vi "LC-MISDK_SimpleInjector.ActivationException.vi"() -> ()   [LabVIEW 2015]
uses:
  C:/Program Files (x86)/National Instruments/LabVIEW 2015/LC-MISDK.dll
  Program Files (x86)/National Instruments/LabVIEW 2015/LC-MISDK.dll
panel:
  out "X":dbl
  out "Y":dbl
  out "Z":dbl
  out "Lv":dbl
  out "Dw":dbl
  out "Pe":dbl
  out "Lv":dbl
  out "Tcp":dbl
  out "Duv":dbl
  out "ReadLatestData Error":dbl format="%#_6f"
  out "Lv":dbl
  out "ud":dbl
  out "vd":dbl
  in  "Get Measurement Data":T1(radio)=enum."Lvxy"
  in  "Measurement":bool
  out "y":dbl
  out "x":dbl
  out "Lv":dbl
  out "Connect error Code":dbl
  in  "EXIT":bool
  in  "Connect":bool
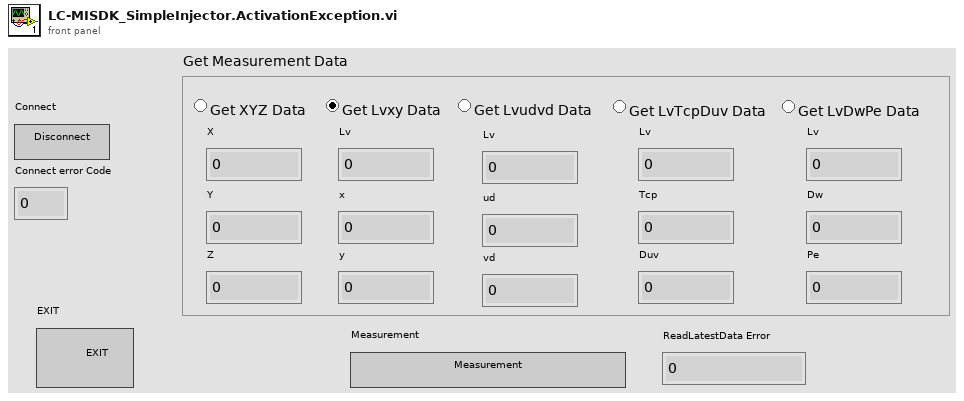
[diagram p1: front panel]
types:
  T1 = enum32{"XYZ", "Lvxy", "Lvudvd", "LvTcpDuv", "LvDwPe"}
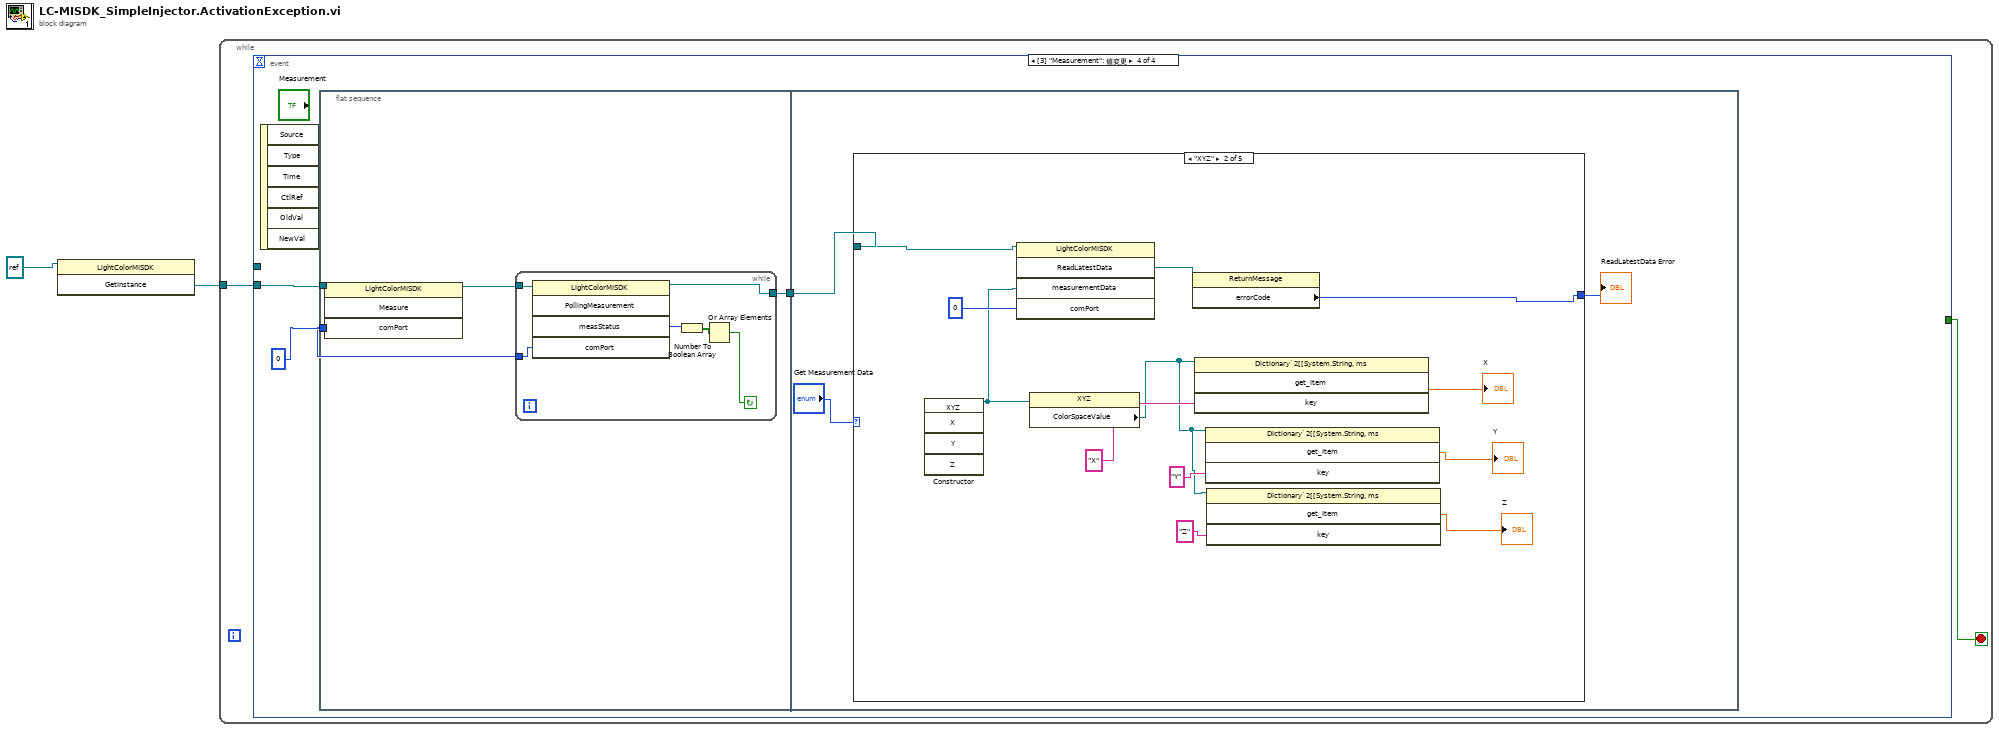
[diagram p0: block diagram]
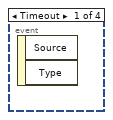
[diagram p2: hidden frame]
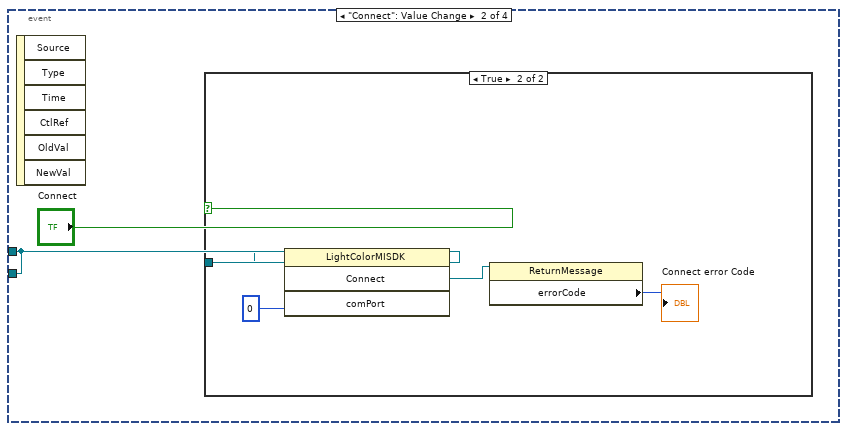
[diagram p3: hidden frame]
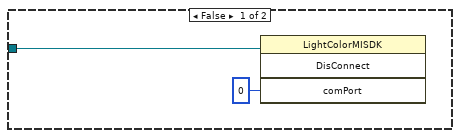
[diagram p4: hidden frame]
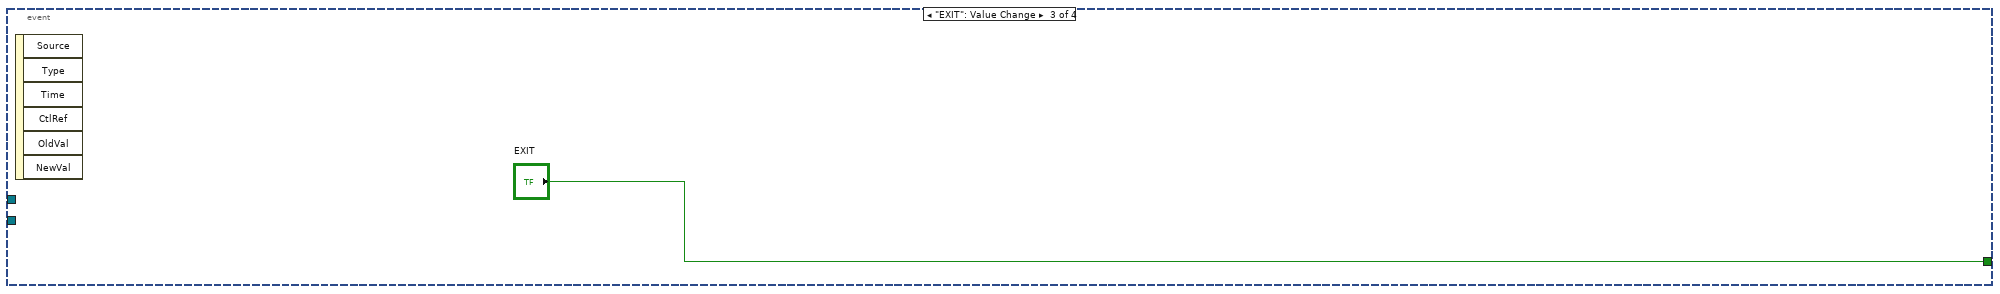
[diagram p5: hidden frame]
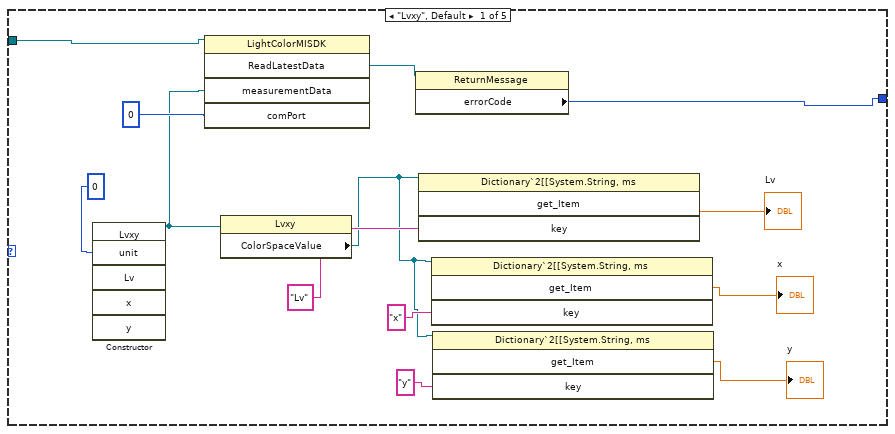
[diagram p6: hidden frame]
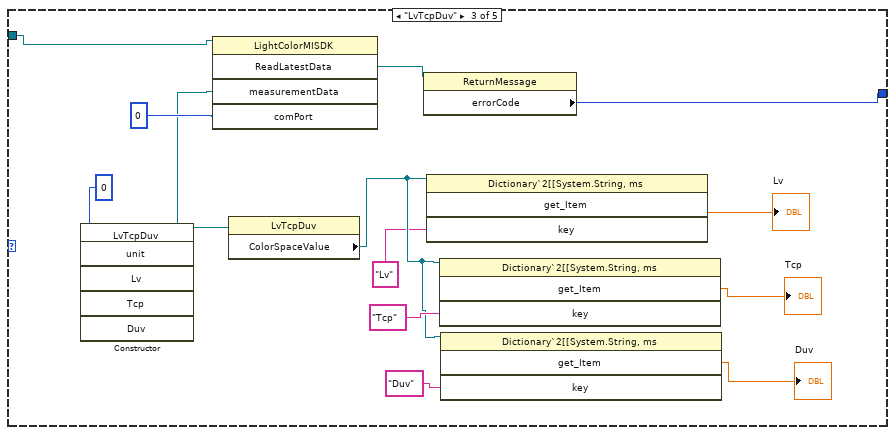
[diagram p7: hidden frame]
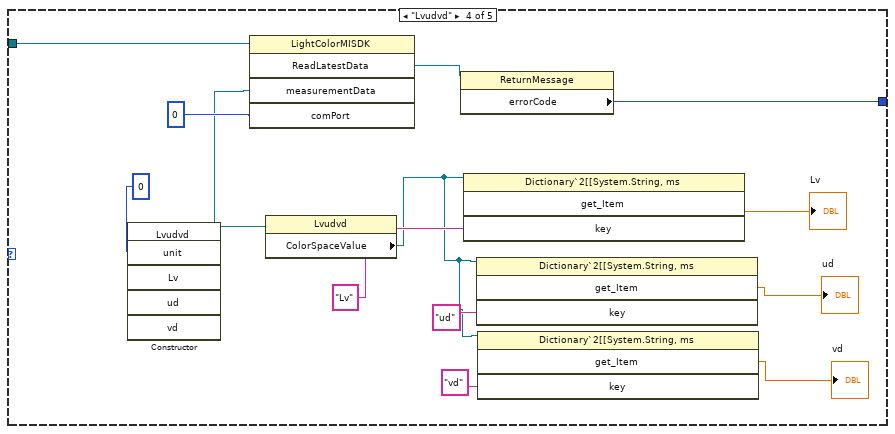
[diagram p8: hidden frame]
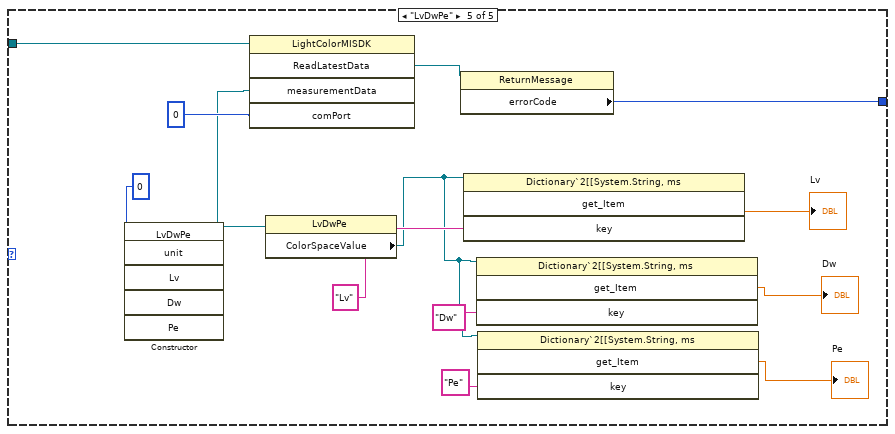
[diagram p9: hidden frame]
diagram:
  n1 = invoke on="インボークノード" class="LightColorMISDK" method="GetInstance"(reference=refnum<k24> refnum ("リファレンス出力")) -> ("GetInstance"=w1:refnum<k24>)  [unwired: 2 in, 2 out]
  n2 = while {
    tunnel: w1 -> [w4]
    stop <- w3 stop-if-true
    n3 = event shown="[3] \"Measurement\": 値変更" {
      selector: _ -> [_ _ _ _]
      dyn-events: _ -> [_ _ _ _]
      timeout: _ -> [_ _ _ _]
      tunnel: [_ w5 _ _] -> _
      tunnel: [_ _ "EXIT" _] -> w3
      tunnel: w4 -> [_ w5 _ w16]
      event Timeout {
        n4 = event-data() -> ()  [unwired: 1 in, 2 out]
      }
      event "Connect": Value Change {
        n5 = event-data() -> ()  [unwired: 1 in, 6 out]
        n6 = case shown="TRUE" "Connect" {
          tunnel: w5 -> [w7 w12]
          frame False {
            n7 = invoke on="インボークノード" class="LightColorMISDK" method="DisConnect"(reference=w7, "comPort"=0) -> ()  [unwired: 2 in, 4 out]
          }
          frame True {
            n8 = invoke on="インボークノード" class="LightColorMISDK" method="Connect"(reference=w12, "comPort"=0) -> ("Connect"=w9:refnum<k24>)  [unwired: 2 in, 3 out]
            n9 = property on="プロパティノード" class="ReturnMessage"(reference=w9) -> ("errorCode"=→"Connect error Code":i32)  [unwired: 1 in, 2 out]
          }
        }
      }
      event "EXIT": Value Change {
        n10 = event-data() -> ()  [unwired: 1 in, 6 out]
      }
      event "Measurement": Value Change {
        n11 = event-data() -> ()  [unwired: 1 in, 6 out]
        n12 = flat-sequence {
          tunnel: w16 -> [w19]
          tunnel: 0 -> [w17]
          tunnel: [w20] -> w14
          tunnel: w14 -> [w28]
          frame #0 {
            n13 = invoke on="インボークノード" class="LightColorMISDK" method="Measure"(reference=w19, "comPort"=w17) -> (reference out=w18:refnum<k24>)  [unwired: 2 in, 3 out]
            n14 = while {
              tunnel: [w25] -> w20
              tunnel: w18 -> [w24]
              tunnel: w17 -> [w23]
              stop <- w21 continue-if-true
              n15 = invoke on="インボークノード" class="LightColorMISDK" method="PollingMeasurement"(reference=w24, "comPort"=w23) -> (reference out=w25:refnum<k24>, "measStatus"=w26:i32)  [unwired: 3 in, 3 out]
              n16 = Number To Boolean Array(number=w26) -> (Boolean array=w22:bool[])
              n17 = Or Array Elements(Boolean array=w22) -> (logical OR=w21:bool)
            }
          }
          frame #1 {
            n18 = case shown="\"XYZ\"" "Get Measurement Data" {
              tunnel: w28 -> [w42 w54 w67 w80 w93]
              tunnel: [w30 w43 w55 w68 w81] -> w27
              frame "Lvxy", Default {
                n19 = constructor class="Lvxy"("unit"=0) -> (reference out=w39:refnum<k24>)  [unwired: 6 in, 6 out]
                n20 = invoke on="インボークノード" class="LightColorMISDK" method="ReadLatestData"(reference=w42, "measurementData"=w39, "comPort"=0) -> ("ReadLatestData"=w40:refnum<k24>)  [unwired: 2 in, 4 out]
                n21 = property class="Lvxy"(reference=w39) -> ("ColorSpaceValue"=w34:refnum<k24>)  [unwired: 1 in, 2 out]
                n22 = property on="プロパティノード" class="ReturnMessage"(reference=w40) -> ("errorCode"=w30:i32)  [unwired: 1 in, 2 out]
                n23 = invoke class="Dictionary`2[[System.String, ms" method="get_Item"(reference=w34, "key"="Lv") -> ("get_Item"=→"Lv":dbl)  [unwired: 2 in, 3 out]
                n24 = invoke class="Dictionary`2[[System.String, ms" method="get_Item"(reference=w34, "key"="x") -> ("get_Item"=→"x":dbl)  [unwired: 2 in, 3 out]
                n25 = invoke class="Dictionary`2[[System.String, ms" method="get_Item"(reference=w34, "key"="y") -> ("get_Item"=→"y":dbl)  [unwired: 2 in, 3 out]
              }
              frame "XYZ" {
                n26 = constructor class="XYZ"() -> (reference out=w51:refnum<k24>)  [unwired: 6 in, 5 out]
                n27 = invoke on="インボークノード" class="LightColorMISDK" method="ReadLatestData"(reference=w54, "measurementData"=w51, "comPort"=0) -> ("ReadLatestData"=w52:refnum<k24>)  [unwired: 2 in, 4 out]
                n28 = property class="XYZ"(reference=w51) -> ("ColorSpaceValue"=w46:refnum<k24>)  [unwired: 1 in, 2 out]
                n29 = property on="プロパティノード" class="ReturnMessage"(reference=w52) -> ("errorCode"=w43:i32)  [unwired: 1 in, 2 out]
                n30 = invoke class="Dictionary`2[[System.String, ms" method="get_Item"(reference=w46, "key"="X") -> ("get_Item"=→"X":dbl)  [unwired: 2 in, 3 out]
                n31 = invoke class="Dictionary`2[[System.String, ms" method="get_Item"(reference=w46, "key"="Y") -> ("get_Item"=→"Y":dbl)  [unwired: 2 in, 3 out]
                n32 = invoke class="Dictionary`2[[System.String, ms" method="get_Item"(reference=w46, "key"="Z") -> ("get_Item"=→"Z":dbl)  [unwired: 2 in, 3 out]
              }
              frame "LvTcpDuv" {
                n33 = constructor class="LvTcpDuv"("unit"=0) -> (reference out=w64:refnum<k24>)  [unwired: 6 in, 6 out]
                n34 = invoke on="インボークノード" class="LightColorMISDK" method="ReadLatestData"(reference=w67, "measurementData"=w64, "comPort"=0) -> ("ReadLatestData"=w65:refnum<k24>)  [unwired: 2 in, 4 out]
                n35 = property class="LvTcpDuv"(reference=w64) -> ("ColorSpaceValue"=w60:refnum<k24>)  [unwired: 1 in, 2 out]
                n36 = property on="プロパティノード" class="ReturnMessage"(reference=w65) -> ("errorCode"=w55:i32)  [unwired: 1 in, 2 out]
                n37 = invoke class="Dictionary`2[[System.String, ms" method="get_Item"(reference=w60, "key"="Lv") -> ("get_Item"=→"Lv":dbl)  [unwired: 2 in, 3 out]
                n38 = invoke class="Dictionary`2[[System.String, ms" method="get_Item"(reference=w60, "key"="Tcp") -> ("get_Item"=→"Tcp":dbl)  [unwired: 2 in, 3 out]
                n39 = invoke class="Dictionary`2[[System.String, ms" method="get_Item"(reference=w60, "key"="Duv") -> ("get_Item"=→"Duv":dbl)  [unwired: 2 in, 3 out]
              }
              frame "Lvudvd" {
                n40 = constructor class="Lvudvd"("unit"=0) -> (reference out=w77:refnum<k24>)  [unwired: 6 in, 6 out]
                n41 = invoke on="インボークノード" class="LightColorMISDK" method="ReadLatestData"(reference=w80, "measurementData"=w77, "comPort"=0) -> ("ReadLatestData"=w78:refnum<k24>)  [unwired: 2 in, 4 out]
                n42 = property class="Lvudvd"(reference=w77) -> ("ColorSpaceValue"=w72:refnum<k24>)  [unwired: 1 in, 2 out]
                n43 = property on="プロパティノード" class="ReturnMessage"(reference=w78) -> ("errorCode"=w68:i32)  [unwired: 1 in, 2 out]
                n44 = invoke class="Dictionary`2[[System.String, ms" method="get_Item"(reference=w72, "key"="Lv") -> ("get_Item"=→"Lv":dbl)  [unwired: 2 in, 3 out]
                n45 = invoke class="Dictionary`2[[System.String, ms" method="get_Item"(reference=w72, "key"="ud") -> ("get_Item"=→"ud":dbl)  [unwired: 2 in, 3 out]
                n46 = invoke class="Dictionary`2[[System.String, ms" method="get_Item"(reference=w72, "key"="vd") -> ("get_Item"=→"vd":dbl)  [unwired: 2 in, 3 out]
              }
              frame "LvDwPe" {
                n47 = constructor class="LvDwPe"("unit"=0) -> (reference out=w90:refnum<k24>)  [unwired: 6 in, 6 out]
                n48 = invoke on="インボークノード" class="LightColorMISDK" method="ReadLatestData"(reference=w93, "measurementData"=w90, "comPort"=0) -> ("ReadLatestData"=w91:refnum<k24>)  [unwired: 2 in, 4 out]
                n49 = property class="LvDwPe"(reference=w90) -> ("ColorSpaceValue"=w85:refnum<k24>)  [unwired: 1 in, 2 out]
                n50 = property on="プロパティノード" class="ReturnMessage"(reference=w91) -> ("errorCode"=w81:i32)  [unwired: 1 in, 2 out]
                n51 = invoke class="Dictionary`2[[System.String, ms" method="get_Item"(reference=w85, "key"="Lv") -> ("get_Item"=→"Lv":dbl)  [unwired: 2 in, 3 out]
                n52 = invoke class="Dictionary`2[[System.String, ms" method="get_Item"(reference=w85, "key"="Dw") -> ("get_Item"=→"Dw":dbl)  [unwired: 2 in, 3 out]
                n53 = invoke class="Dictionary`2[[System.String, ms" method="get_Item"(reference=w85, "key"="Pe") -> ("get_Item"=→"Pe":dbl)  [unwired: 2 in, 3 out]
              }
            }
            "ReadLatestData Error" <- w27
          }
        }
      }
    }
  }
